vi "get_img_info.vi"(4 "LabVIEW Web Service Request":refnum<class "Web Request.lvclass">) -> ()   [LabVIEW 2015]
uses:
  <vilib>/wsapi/Web Request.lvclass
  global_cms.vi
panel:
  # "Use the Web Service Request input terminal to call the VIs on the Web Services palette. Do not remove it from the connector pane unless you don't need access to the palette."
  # "Each additional control wired to the connector pane will be available as an input in the URL. To include an indicator in terminal-mode output (the default setting), it must also be wired to the connector pane."
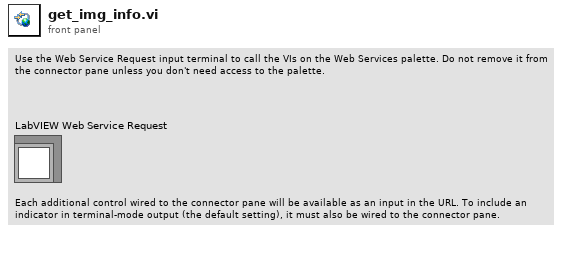
[diagram p1: front panel]
types:
  T1 = cluster{"data":cluster{"fileRequest":cluster{"filePath":string, "fileType":string, "fileName":string, "time":u32, "filePathTmp":string, "fileSize":u32}, "fileResponse":cluster{"filePath":string, "fileType":string, "fileName":string, "decode":string, "result":string, "status":string, "time":u32, "size":u32}}[], "_status":string, "_token":string}
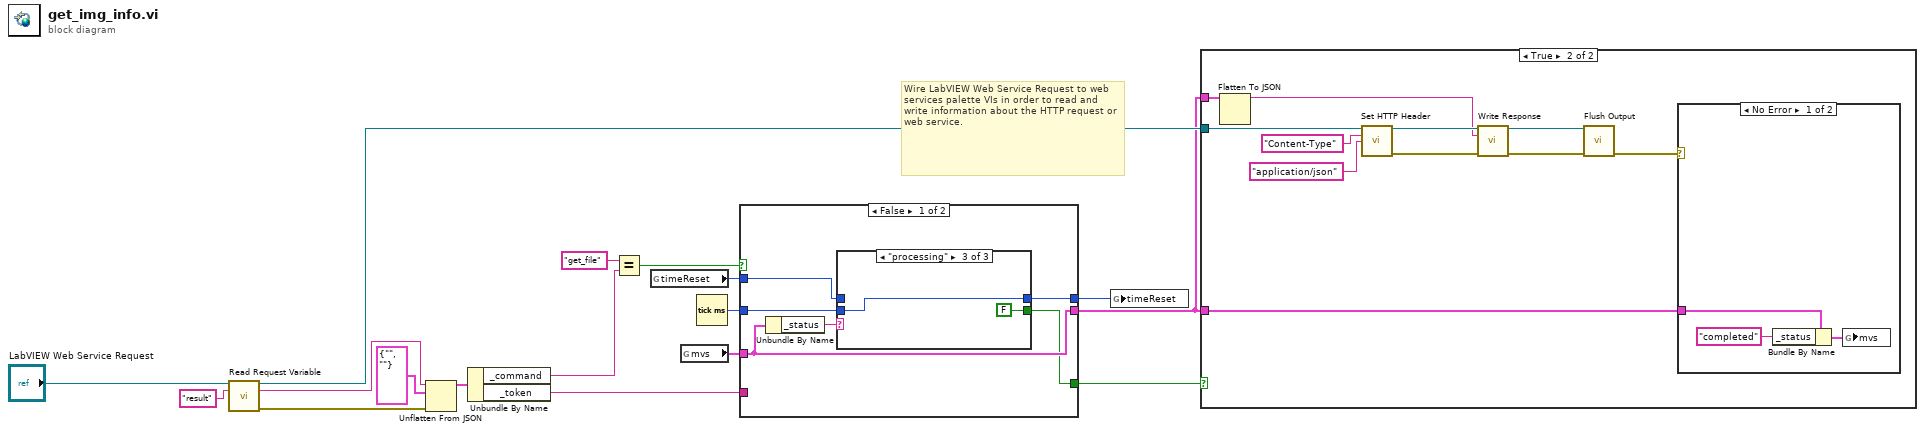
[diagram p0: block diagram]
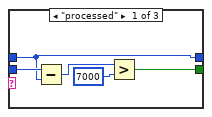
[diagram p4: hidden frame]
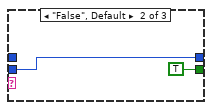
[diagram p5: hidden frame]
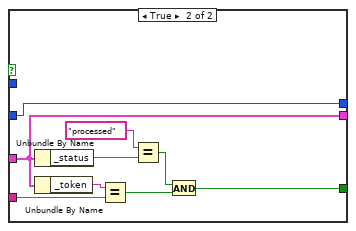
[diagram p6: hidden frame]
diagram:
  # "Wire LabVIEW Web Service Request to web services palette VIs in order to read and write information about the HTTP request or web service."
  n1 = call <vilib>:"Read Request Variable.vi"("LabVIEW Web Service Request"="LabVIEW Web Service Request", "variable name"="result" ("key")) -> ("LabVIEW Web Service Request out"=w5:refnum<class "Web Request.lvclass">, "value"=w14:string, "error out"=w13:errorcluster)  [unwired: 11 in]
  n2 = Unflatten From JSON(JSON string=w14, type and defaults=cluster{"_command":string, "_token":string} {"_command"="", "_token"=""}, error in (no error)=w13) -> (value=w12:cluster{"_command":string, "_token":string})  [unwired: 4 in, 1 out]
  n3 = Unbundle By Name(w12) -> ("_command"=w10:string, "_token"=w9:string)
  n4 = Equal?(x="get_file", y=w10) -> (x = y?=w8:bool)
  n5 = global read "global_cms.vi" "timeReset"() -> (w3:u32)
  n6 = global read "global_cms.vi" "mvs"() -> (w7:T1)
  n7 = Tick Count (ms)() -> (millisecond timer value=w1:u32)
  n8 = case shown="False" w8 {
    tunnel: w9 -> [_ w41]
    tunnel: w7 -> [w23 w35]
    tunnel: [w21 w34] -> w6
    tunnel: [w23 w35] -> w4
    tunnel: w3 -> [w20 _]
    tunnel: [w19 w33] -> w2
    tunnel: w1 -> [w18 w33]
    frame False {
      n9 = Unbundle By Name(w23) -> ("_status"=w22:string)
      n10 = case shown="\"processing\"" w22 {
        tunnel: [w28 TRUE FALSE] -> w21
        tunnel: w20 -> [w24 _ _]
        tunnel: [w24 w29 w31] -> w19
        tunnel: w18 -> [w25 w29 w31]
        frame "processed" {
          n11 = Subtract(x=w25, y=w24) -> (x-y=w27:u32)
          n12 = Greater?(x=w27, y=u32 7000) -> (0:w28:bool)
        }
        frame "False", Default {
        }
        frame "processing" {
        }
      }
    }
    frame True {
      n13 = Unbundle By Name(w35) -> ("_status"=w39:string)
      n14 = Unbundle By Name(w35) -> ("_token"=w40:string)
      n15 = Equal?(x=w40, y=w41) -> (x = y?=w36:bool)
      n16 = Equal?(x="processed", y=w39) -> (x = y?=w37:bool)
      n17 = And(x=w37, y=w36) -> (x .and. y?=w34:bool)
    }
  }
  n18 = global write "global_cms.vi" "timeReset"(w2) -> ()
  n19 = case shown="True" w6 {
    tunnel: w4 -> [_ w45]
    tunnel: w5 -> [_ w44]
    tunnel: w4 -> [_ w42]
    frame False {
    }
    frame True {
      n20 = Flatten To JSON(anything=w45) -> (JSON string=w47:string)  [unwired: 2 in, 1 out]
      n21 = call <vilib>:"Set HTTP Header.vi"("LabVIEW Web Service Request"=w44, "header"="Content-Type", "header value"="application/json") -> ("LabVIEW Web Service Request out"=w48:refnum<class "Web Request.lvclass">, "error out"=w46:errorcluster)  [unwired: 11 in]
      n22 = call <vilib>:"Write Response.vi"("LabVIEW Web Service Request"=w48, "response string"=w47, "error in (no error)"=w46) -> ("LabVIEW Web Service Request out"=w50:refnum<class "Web Request.lvclass">, "error out"=w49:errorcluster)  [unwired: 11 in]
      n23 = call <vilib>:"Flush Output.vi"("LabVIEW Web Service Request"=w50, "error in (no error)"=w49) -> ("error out"=w43:errorcluster)  [unwired: 12 in, 1 out]
      n24 = case shown="No Error" w43 {
        tunnel: w42 -> [w55 _]
        frame No Error {
          n25 = Bundle By Name(cluster=w55, "_status"="completed") -> (w53:T1)
          n26 = global write "global_cms.vi" "mvs"(w53) -> ()
        }
        frame Error {
        }
      }
    }
  }
